vi "Query.vi"(0 "reference in":refnum<class "Database_ODBC.lvclass">, 5 "Query":string, 7 "Timeout":i32=10000, 11 "error in (no error)":errorcluster) -> (4 "reference out":refnum<class "Database_ODBC.lvclass">, 6 "Query Return":T1[](array[typedef]), 15 "error out":errorcluster)   [LabVIEW 2019, in "Database_ODBC.lvclass"]
uses:
  Database_ODBC.lvclass
  Database_Postgress_class/Query Return.ctl
  Database_ODBC.lvclass/Database_ODBC.ctl
  <vilib>/addons/database/Connection.llb/Conn Execute.vi
  <vilib>/addons/database/Recordset.llb/Rec Fetch Recordset Data (R).vi
  <vilib>/addons/database/_DB Variant To Data/Database Variant To Data.xnode
  <vilib>/addons/database/NI_Database_API.lvlib
  DatabaseInterface_class/DatabaseInterface.lvclass
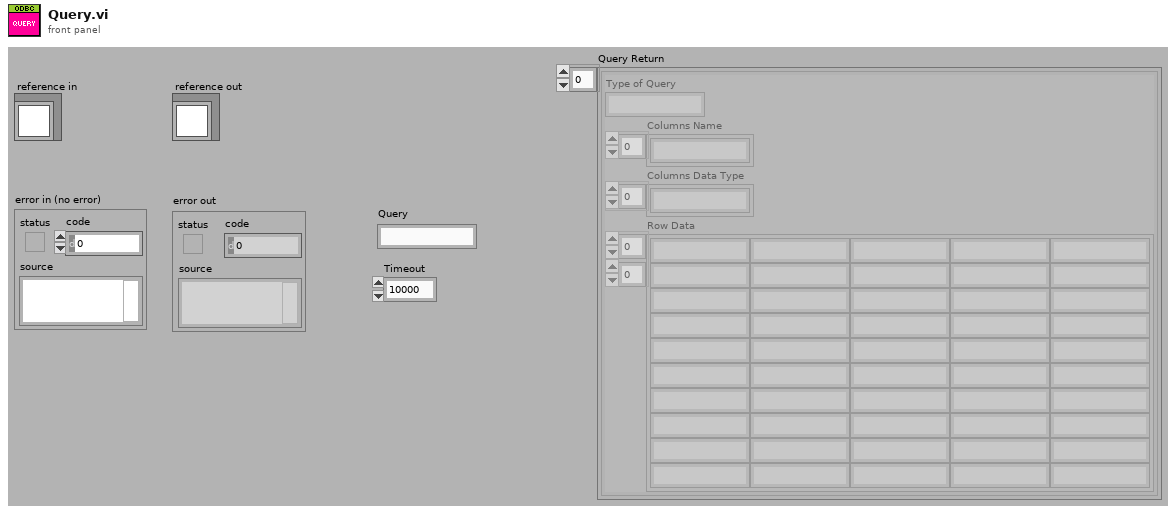
[diagram p1: front panel]
types:
  T1 = typedef "DatabaseInterface.lvclass/Query Return.ctl" = cluster{"Type of Query":string, "Columns Name":string[], "Columns Data Type":string[], "Row Data":string[][]}
  T2 = typedef "NI_Database_API.lvlib/Conn ObjectReference.ctl" = refnum<k1>
  T3 = typedef "NI_Database_API.lvlib/Rec ObjectReference.ctl" = refnum<k1>
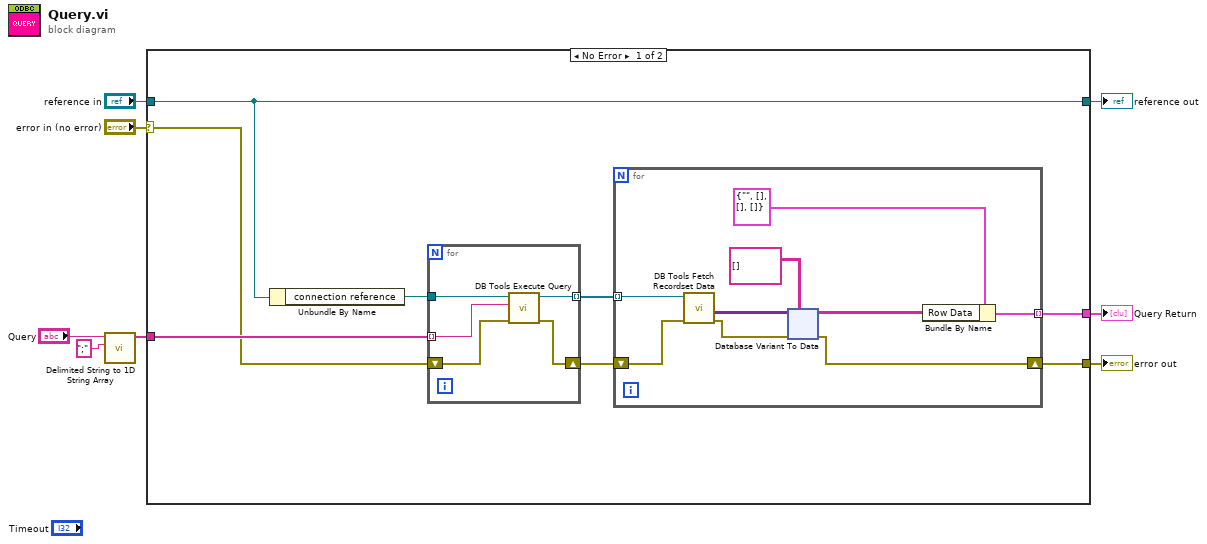
[diagram p0: block diagram]
diagram:
  n1 = call <vilib>:"Delimited String to 1D String Array.vi"("delimiter"=";", "delimited string"="Query") -> ("string array"=w2:string[])  [unwired: 9 in]
  n2 = case shown="No Error" "error in (no error)" {
    selector: "error in (no error)" -> [w14 w76]
    tunnel: [w11 w76] -> w7
    tunnel: [w9 w75] -> w5
    tunnel: "reference in" -> [w9 w75]
    tunnel: w2 -> [w15 _]
    tunnel: [w10 _] -> w1
    frame No Error {
      n3 = Unbundle By Name(w9) -> ("connection reference"=w16:T2)
      n4 = for {
        tunnel: w16 -> [w74]
        tunnel: w15 -> [w73] mode=indexing
        tunnel: [w72] -> w13 mode=indexing
        shift-right: [w71] -> w12
        shift-left: w14 -> [w70]
        n5 = call-poly <vilib>:"DB Tools Execute Query.vi"("error in (no error)"=w70, "SQL query"=w73, "connection reference"=w74) -> ("error out"=w71:errorcluster, "recordset reference"=w72:T3)  [unwired: 5 in]
      }
      n6 = for {
        tunnel: w13 -> [w25] mode=indexing
        shift-right: [w21] -> w11
        shift-left: w12 -> [w24]
        tunnel: [w17] -> w10 mode=indexing
        n7 = call-poly <vilib>:"DB Tools Fetch Recordset Data.vi"("error in (no error)"=w24, "recordset reference"=w25) -> ("error out"=w22:errorcluster, "recordset data"=w23:variant[][])  [unwired: 3 in, 1 out]
        n8 = xnode "Database Variant To Data"("database variant"=w23, "error in (no error)"=w22, "type"=string[][] []) -> ("data"=w18:string[][], "error out"=w21:errorcluster)
        n9 = Bundle By Name(cluster=T1 {"Type of Query"="", "Columns Name"=[], "Columns Data Type"=[], "Row Data"=[]} ("Query Return"), "Row Data"=w18) -> (w17:T1)
      }
    }
    frame Error {
    }
  }
  "error out" <- w7
  "reference out" <- w5
  "Query Return" <- w1
